vi "HEWH RLT Read Channels Multi.vi"(8 "Error In":errorcluster, 10 "Raw Data Input":string[][](array[string]), 11 "Panel Input":T1[][](array[typedef])) -> (0 "Error Out":errorcluster, 1 "Panel 3":T1[][](array[typedef]), 2 "Panel 2":T1[][](array[typedef]), 3 "Panel 1":T1[][](array[typedef]))   [LabVIEW 2016]
uses:
  Type Definitions/HEWH Channel Label RLT.ctl
  Custom Instrument Control/MW100/Type Definitions/Station ID Selector.ctl
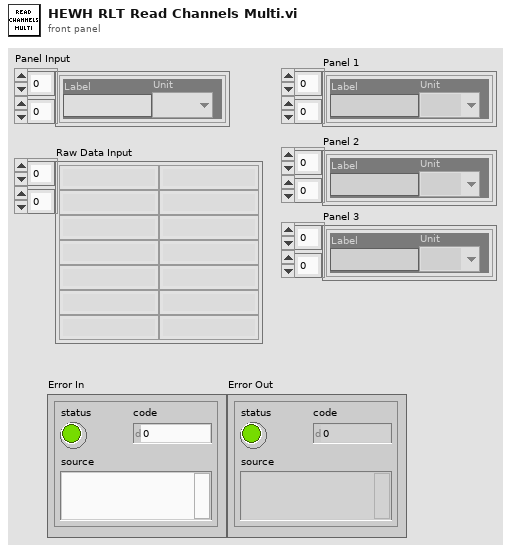
[diagram p1: front panel]
types:
  T1 = typedef "HEWH Channel Label RLT.ctl" = cluster{"Label":string, "Unit":T2}
  T2 = typedef "Station ID Selector.ctl" = enum16{"", "A", "B", "C", "D", "Global"}
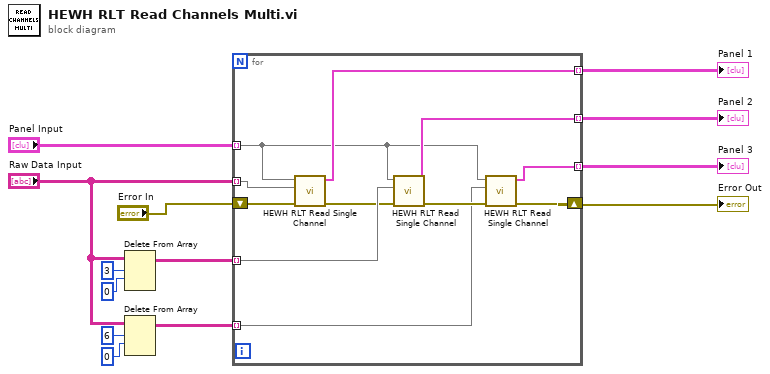
[diagram p0: block diagram]
diagram:
  n1 = Delete From Array(array="Raw Data Input", length=3, index (row)=0) -> (array with subset deleted=w7:string[][])  [unwired: 1 in, 1 out]
  n2 = Delete From Array(array="Raw Data Input", length=6, index (row)=0) -> (array with subset deleted=w11:string[][])  [unwired: 1 in, 1 out]
  n3 = for {
    tunnel: "Panel Input" -> [w20] mode=indexing
    tunnel: "Raw Data Input" -> [w22] mode=indexing
    tunnel: [w21] -> w4 mode=indexing
    tunnel: w7 -> [w24] mode=indexing
    tunnel: w11 -> [w14] mode=indexing
    tunnel: [w23] -> w12 mode=indexing
    tunnel: [w19] -> w13 mode=indexing
    shift-right: [w15] -> w1
    shift-left: "Error In" -> [w16]
    n4 = call "HEWH RLT Read Single Channel.vi"("Error In"=w16, "all rows"=w22, "Panel In"=w20) -> ("Error Out"=w18:errorcluster, "Panel Out"=w21:T1[])  [unwired: 7 in]
    n5 = call "HEWH RLT Read Single Channel.vi"("Error In"=w18, "all rows"=w24, "Panel In"=w20) -> ("Error Out"=w17:errorcluster, "Panel Out"=w23:T1[])  [unwired: 7 in]
    n6 = call "HEWH RLT Read Single Channel.vi"("Error In"=w17, "all rows"=w14, "Panel In"=w20) -> ("Error Out"=w15:errorcluster, "Panel Out"=w19:T1[])  [unwired: 7 in]
  }
  "Panel 3" <- w13
  "Panel 2" <- w12
  "Panel 1" <- w4
  "Error Out" <- w1
